vi "SetUSB2AiRange.vi"(8 "Range":sgl=10.0, 11 "error in":errorcluster caption="错误输入") -> (3 "error out":errorcluster caption="错误输出")   [LabVIEW 2016]
uses:
  PLC-Lab/lib/gusb.dll
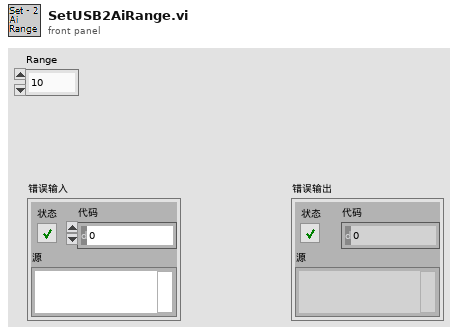
[diagram p1: front panel]
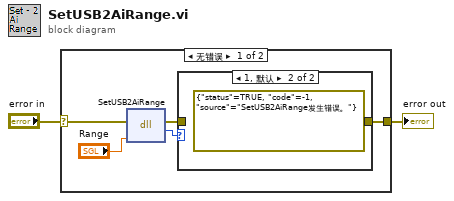
[diagram p0: block diagram]
diagram:
  n1 = case shown="无错误" "error in" {
    selector: "error in" -> [w7 w10]
    tunnel: [w4 w10] -> w1
    frame No Error {
      n2 = dll-call lib="E:/Camproject/2018/2018.1Labview/PLC-Lab/lib/gusb.dll" fn="SetUSB2AiRange"(error in=w7, "Range"="Range") -> (error out=w5:errorcluster, "Status"=w6:i32)  [unwired: 3 in, 1 out]
      n3 = case shown="1, 默认" w6 {
        tunnel: w5 -> [w8 _]
        tunnel: [w8 errorcluster {"status"=TRUE, "code"=-1, "source"="SetUSB2AiRange发生错误。"} ("错误常量")] -> w4
        frame 0 {
        }
        frame 1, Default {
        }
      }
    }
    frame Error {
    }
  }
  "error out" <- w1
